vi "Initialize.vi"(8 "error in":errorcluster, 11 "Plugin in":refnum<class "Sequencer with Output Values.lvclass">) -> (0 "error out":errorcluster, 3 "Plugin out":refnum<class "Sequencer with Output Values.lvclass">)   [LabVIEW 2024, in "Sequencer with Output Values.lvlib" / "Sequencer with Output Values.lvclass"]
uses:
  Sequencer with Output Values.lvclass
  C:/Program Files/National Instruments/LabVIEW 2024/vi.lib/FlexLogger/SDK/PluginSDK.lvlibp/PEFClasses/SDK/Plugin/Plugin.lvclass
  <vilib>/FlexLogger/SDK/PluginSDK.lvlibp/PEFClasses/SDK/Processing Element/Timing Parameters.ctl
  <vilib>/FlexLogger/SDK/PluginSDK.lvlibp/PEFClasses/SDK/Processing Element/Timing Method.ctl
  Params.ctl
  Step Settings.ctl
  Sequencer with Output Values.lvclass/Sequencer with Output Values.ctl
  <vilib>/FlexLogger/SDK/PluginSDK.lvlibp/PEFClasses/SDK/Producer Channel/Producer Channel.lvclass
  C:/Program Files/National Instruments/LabVIEW 2024/vi.lib/FlexLogger/SDK/PluginSDK.lvlibp/PEFClasses/SDK/Channel/Channel.lvclass
  Global Strings.vi
  <vilib>/FlexLogger/SDK/PluginSDK.lvlibp/PEFClasses/SDK/Plugin/ParameterAccess/Write Command.vi
  <vilib>/FlexLogger/SDK/PluginSDK.lvlibp/PEFClasses/SDK/Plugin/ParameterAccess/Read String.vi
  <vilib>/FlexLogger/SDK/PluginSDK.lvlibp/PEFClasses/SDK/Plugin/ParameterAccess/Write String.vi
  Settings UI.vi
  <vilib>/FlexLogger/SDK/PluginSDK.lvlibp/PEFClasses/SDK/Producer Channel/Create Producer Channel.vi
  <vilib>/FlexLogger/SDK/PluginSDK.lvlibp/PEFClasses/SDK/Plugin/Plugin.lvclass
  <vilib>/FlexLogger/SDK/PluginSDK.lvlibp/PEFClasses/SDK/Processing Element/Processing Element.lvclass
  <vilib>/FlexLogger/SDK/PluginSDK.lvlibp
  C:/Program Files/National Instruments/LabVIEW 2024/vi.lib/FlexLogger/SDK/PluginSDK.lvlibp/PEFClasses/SDK/Processing Element/Processing Element.lvclass
  C:/dev/niflexlogger-plugins/plugins/Sequencer with Output Values/source/Sequencer with Output Values/Sequencer with Output Values.lvclass
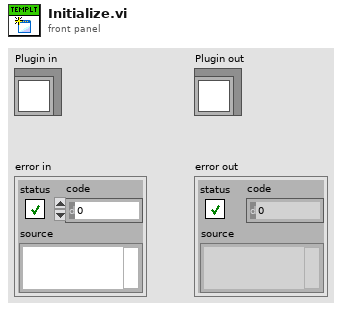
[diagram p1: front panel]
types:
  T1 = typedef "Sequencer with Output Values.lvlib/Sequencer with Output Values.lvclass/Step Settings.ctl" = cluster{"Duration":dbl, "Mode":string, "Delay Between Values":dbl, "Analog Values":string[], "Digital Values":string[]}
  T2 = typedef "Sequencer with Output Values.lvlib/Sequencer with Output Values.lvclass/Params.ctl" = cluster{"Step Values":T1[], "Only Execute When Test Running":bool, "Reset Sequence When Test Starts":bool, "Current Sequence ID":u32, "Total Iterations":u32, "Last Timestamp":dbl, "Number of Sequence Steps":i32, "Num of Analog Channels":i32, "Num of Digital Channels":i32, "Delay Before Starting Sequence":dbl, "Changed":bool}
  T3 = typedef "PluginSDK.lvlibp/Processing Element.lvclass/Timing Parameters.ctl" = cluster{"Timing Method":T4, "Timing Period (ms)":i32}
  T4 = typedef "PluginSDK.lvlibp/Processing Element.lvclass/Timing Method.ctl" = enum16{"Periodic", "Immediate", "On Data Ready", "Triggered"}
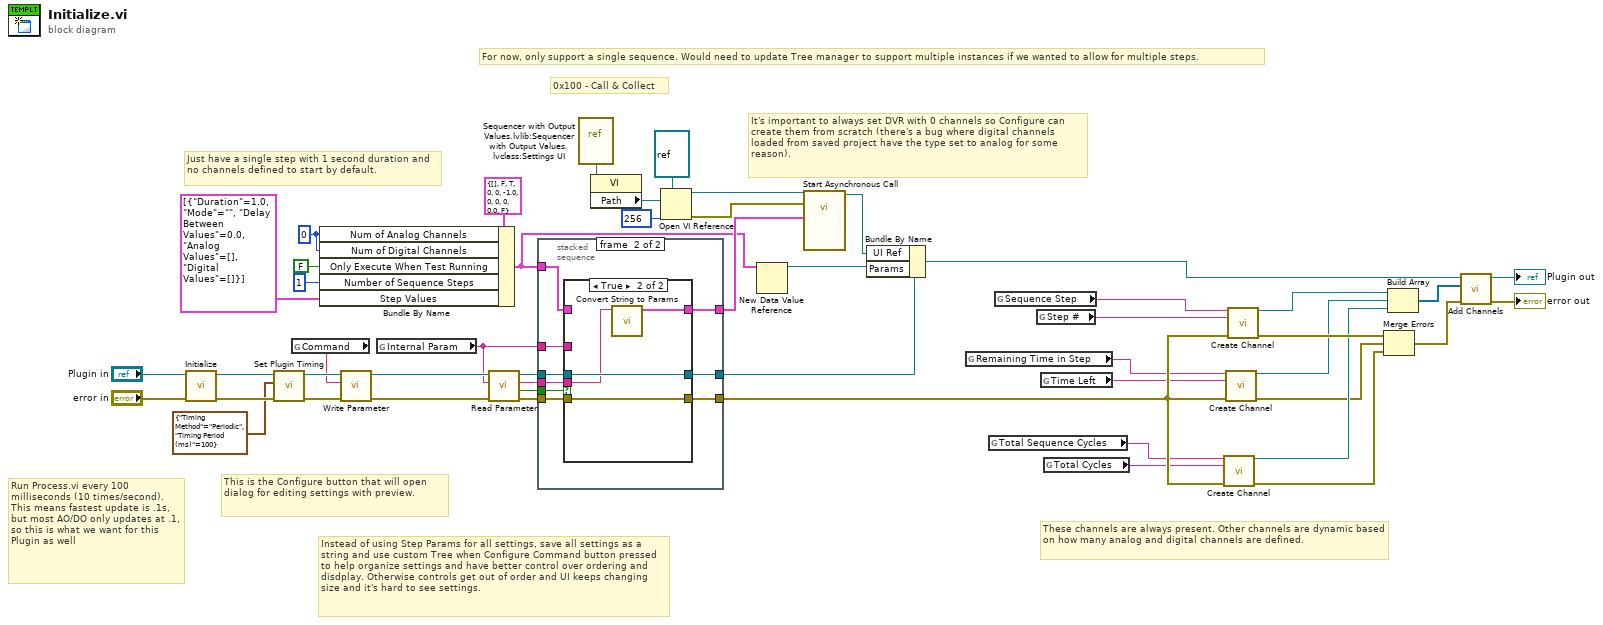
[diagram p0: block diagram]
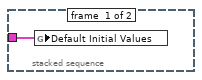
[diagram p2: hidden frame]
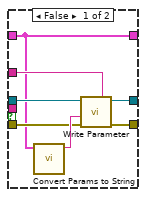
[diagram p3: hidden frame]
diagram:
  w17 = 0 ("Num of Analog Channels")
  # "For now, only support a single sequence. Would need to update Tree manager to support multiple instances if we wanted to allow for multiple steps."
  # "0x100 - Call & Collect"
  # "It's important to always set DVR with 0 channels so Configure can create them from scratch (there's a bug where digital channels loaded from saved project have the type set to analog for some reason)."
  # "This is the Configure button that will open dialog for editing settings with preview."
  # "Instead of using Step Params for all settings, save all settings as a string and use custom Tree when Configure Command button pressed to help organize settings and have better control over ordering and disdplay. Otherwise controls get out of order and UI keeps changing size and it's hard to see settings."
  # "Just have a single step with 1 second duration and no channels defined to start by default."
  # "These channels are always present. Other channels are dynamic based on how many analog and digital channels are defined."
  # "Run Process.vi every 100 milliseconds (10 times/second). This means fastest update is .1s, but most AO/DO only updates at .1, so this is what we want for this Plugin as well"
  n1 = call-parent "Initialize.vi"("error in (no error)"="error in", "Plugin in"="Plugin in") -> ("error out"=w47:errorcluster, "Plugin out"=w45:refnum<class "Sequencer with Output Values.lvclass">)  [unwired: 8 in]
  n2 = call <vilib>:"Set Plugin Timing.vi"("error in (no error)"=w47, "Timing Parameters"=T3 {"Timing Method"=enum."Periodic", "Timing Period (ms)"=100}, "Plugin in"=w45) -> ("error out"=w31:errorcluster, "Plugin out"=w32:refnum<class "Sequencer with Output Values.lvclass">)  [unwired: 7 in]
  n3 = global read "Global Strings.vi" "Command"() -> (w30:string)
  n4 = Bundle By Name(cluster=T2 {"Step Values"=[], "Only Execute When Test Running"=FALSE, "Reset Sequence When Test Starts"=TRUE, "Current Sequence ID"=0, "Total Iterations"=0, "Last Timestamp"=-1.0, "Number of Sequence Steps"=0, "Num of Analog Channels"=0, "Num of Digital Channels"=0, "Delay Before Starting Sequence"=0.0, "Changed"=FALSE}, "Num of Analog Channels"=w17, "Num of Digital Channels"=w17, "Only Execute When Test Running"=FALSE, "Number of Sequence Steps"=1, "Step Values"=T1[] [{"Duration"=1.0, "Mode"="", "Delay Between Values"=0.0, "Analog Values"=[], "Digital Values"=[]}]) -> (w10:T2)
  n5 = call-poly <vilib>:"Write Parameter.vi"("error in (no error)"=w31, "Name"=w30, "Plugin in"=w32) -> ("error out"=w23:errorcluster, "Plugin out"=w24:refnum<class "Sequencer with Output Values.lvclass">)  [unwired: 7 in]
  n6 = global read "Global Strings.vi" "Internal Param"() -> (w20:string)
  n7 = call-poly <vilib>:"Read Parameter.vi"("error in (no error)"=w23, "Name"=w20, "Plugin in"=w24) -> ("error out"=w21:errorcluster, "Found"=w19:bool, "Value"=w18:string, "Plugin out"=w22:refnum<class "Sequencer with Output Values.lvclass">)  [unwired: 5 in]
  n8 = stacked-sequence {
    tunnel: [_ w59] -> w27
    tunnel: [_ w58] -> w26
    tunnel: w22 -> [_ w57]
    tunnel: w21 -> [_ w56]
    tunnel: w20 -> [_ w55]
    tunnel: w19 -> [_ w54]
    tunnel: w18 -> [_ w53]
    tunnel: [_ w52] -> w15
    tunnel: w10 -> [w50 w51]
    frame #0 {
      n9 = global write "Global Strings.vi" "Default Initial Values"(w50) -> ()
    }
    frame #1 {
      n10 = case shown="True" w54 {
        tunnel: w51 -> [w60 _]
        tunnel: [w65 w69] -> w59
        tunnel: [w64 w70] -> w58
        tunnel: w57 -> [w63 w70]
        tunnel: w56 -> [w62 w69]
        tunnel: w55 -> [w61 _]
        tunnel: w53 -> [_ w68]
        tunnel: [w60 w67] -> w52
        frame False {
          n11 = call "Convert Params to String.vi"("Settings"=w60) -> ("String out"=w66:string)  [unwired: 10 in]
          n12 = call-poly <vilib>:"Write Parameter.vi"("error in (no error)"=w62, "Value"=w66, "Name"=w61, "Plugin in"=w63) -> ("error out"=w65:errorcluster, "Plugin out"=w64:refnum<class "Sequencer with Output Values.lvclass">)  [unwired: 6 in]
        }
        frame True {
          n13 = call "Convert String to Params.vi"("String In"=w68) -> ("Param Out"=w67:T2)  [unwired: 9 in, 1 out]
        }
      }
    }
  }
  n14 = vi-ref "Sequencer with Output Values.lvlib:Sequencer with Output Values.lvclass:Settings UI.vi"() -> (w12:refnum<vi>)
  n15 = property class="VI"(reference=w12) -> ("Path"=w11:path)  [unwired: 1 in, 2 out]
  n16 = Open VI Reference(type specifier VI Refnum (for type only)=refnum<vi> refnum, vi path=w11, options=256) -> (vi reference=w14:refnum<vi>, error out=w13:errorcluster)  [unwired: 3 in]
  n17 = New Data Value Reference(data value=w10) -> (data value reference=w3:refnum<data-value>)  [unwired: 1 in, 1 out]
  n18 = call-by-ref "Start Asynchronous Call"(reference=w14, error in=w13, "Settings In"=w15) -> (reference out=w1:refnum<vi>)  [unwired: 11 in, 1 out]
  n19 = Bundle By Name(cluster=w26, "UI Ref"=w1, "Params"=w3) -> (w25:refnum<class "Sequencer with Output Values.lvclass">)
  n20 = global read "Global Strings.vi" "Remaining Time in Step"() -> (w7:string)
  n21 = global read "Global Strings.vi" "Total Sequence Cycles"() -> (w5:string)
  n22 = global read "Global Strings.vi" "Sequence Step"() -> (w9:string)
  n23 = global read "Global Strings.vi" "Step #"() -> (w8:string)
  n24 = global read "Global Strings.vi" "Time Left"() -> (w6:string)
  n25 = global read "Global Strings.vi" "Total Cycles"() -> (w4:string)
  n26 = call-poly <vilib>:"Create Channel.vi"("Unique Channel Identifier"=w5, "Default Channel Name"=w4, "error in (no error)"=w27) -> ("Producer Channel"=w38:refnum<class "Producer Channel.lvclass">, "error out"=w36:errorcluster)  [unwired: 11 in]
  n27 = call-poly <vilib>:"Create Channel.vi"("Unique Channel Identifier"=w7, "Default Channel Name"=w6, "error in (no error)"=w27) -> ("Producer Channel"=w39:refnum<class "Producer Channel.lvclass">, "error out"=w37:errorcluster)  [unwired: 11 in]
  n28 = call-poly <vilib>:"Create Channel.vi"("Unique Channel Identifier"=w9, "Default Channel Name"=w8, "error in (no error)"=w27) -> ("Producer Channel"=w40:refnum<class "Producer Channel.lvclass">, "error out"=w41:errorcluster)  [unwired: 11 in]
  n29 = Merge Errors(w41, w37, w36) -> (w43:errorcluster)
  n30 = Build Array(w40, w39, w38) -> (w44:refnum<class "Producer Channel.lvclass">[])
  n31 = call <vilib>:"Add Channels.vi"("error in (no error)"=w43, "Channels"=w44, "Plugin in"=w25) -> ("error out"=→"error out":errorcluster, "Plugin out"=→"Plugin out":refnum<class "Sequencer with Output Values.lvclass">)  [unwired: 7 in]
